vi "Actor Core.vi"(8 "error in":errorcluster, 11 "Image Acquisition in":refnum<class "Image Acquisition.lvclass">) -> (0 "error out":errorcluster, 3 "Actor out":refnum<class "Actor.lvclass">)   [LabVIEW 2016, in "Image Acquisition.lvlib" / "Image Acquisition.lvclass"]
doc: "(<B>Filename</B>: Actor Framework.lvlib:Actor.lvclass:Actor Core.vi)\n\nReceives messages to the actor, reacts to them, and initiates any error handling that may shut the actor down.\n\nDescendant classes may override this VI to append parallel tasks for the actor to complete while it handles messages. Overrides use the Call Parent Method node."
uses:
  Image Acquisition.lvclass
  C:/Program Files (x86)/National Instruments/LabVIEW 2016/vi.lib/ActorFramework/Actor/Actor.lvclass
  <vilib>/ActorFramework/Actor/Actor.lvclass
  Controls/States.ctl
  Controls/Acuisition Actor Data.ctl
  UI/UI/Controls/Start Acquisition.ctl
  <vilib>/userdefined/High Color/IMAQdx.ctl
  <vilib>/ActorFramework/Message Enqueuer/Message Enqueuer.lvclass
  <vilib>/vision/Image Controls.llb/IMAQ Image.ctl
  Image Acquisition.lvclass/Image Acquisition.ctl
  <vilib>/ActorFramework/Actor/Actor.lvclass/Actor.ctl
  <vilib>/ActorFramework/Message Enqueuer/Message Enqueuer.lvclass/Message Enqueuer.ctl
  Image Acquisition Messages/UpdatedMethod Msg/UpdatedImage Msg.lvclass/UpdatedImage Msg.ctl
  <vilib>/ActorFramework/Message Enqueuer/Init from Existing Queue.vi
  <vilib>/ActorFramework/Message Enqueuer/Enqueue.vi
  Image Acquisition Messages/UpdatedMethod Msg/UpdatedImage Msg.lvclass
  C:/Program Files (x86)/National Instruments/LabVIEW 2016/vi.lib/ActorFramework/Message/Message.lvclass
  <vilib>/ActorFramework/Stop Msg/Stop Msg.lvclass
  <vilib>/ActorFramework/Message Priority Queue/Priority Enqueue.vi
  <vilib>/vision/driver/NI_Vision_Acquisition_Software.lvlib
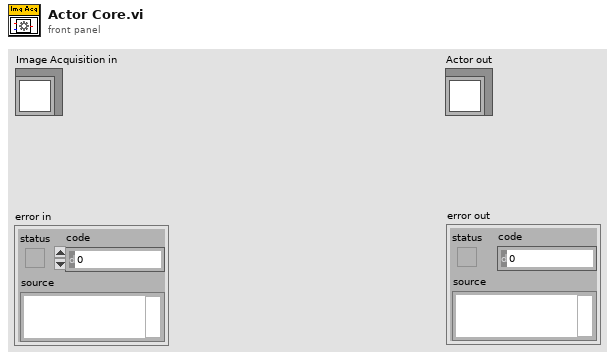
[diagram p1: front panel]
types:
  T1 = typedef "Acuisition Actor Data.ctl" = cluster{"Start Acquisition":T2, "Caller Enqueuer":refnum<class "Message Enqueuer.lvclass">, "Self Enqueuer":refnum<class "Message Enqueuer.lvclass">, "UI Enqueuer":refnum<class "Message Enqueuer.lvclass">, "Image Acquisition in":refnum<class "Image Acquisition.lvclass">, "Target Actor Enqueuer":refnum<class "Message Enqueuer.lvclass">, "Live Session":T3, "Live Image Buffer":T4, "Started?":bool}
  T2 = typedef "Start Acquisition.ctl" = cluster{"Image Indicator Reference":refnum<vi>, "Start":bool, "Camera":T3}
  T3 = typedef "IMAQdx.ctl" = refnum<k21>
  T4 = typedef "IMAQ Image.ctl" = refnum<image>
  T5 = typedef "States.ctl" = enum16{"Poll", "Initialize", "Start Acquisition", "Snap Image", "Stop Acquistion", "Error"}
  T6 = typedef "Image Type" = u32
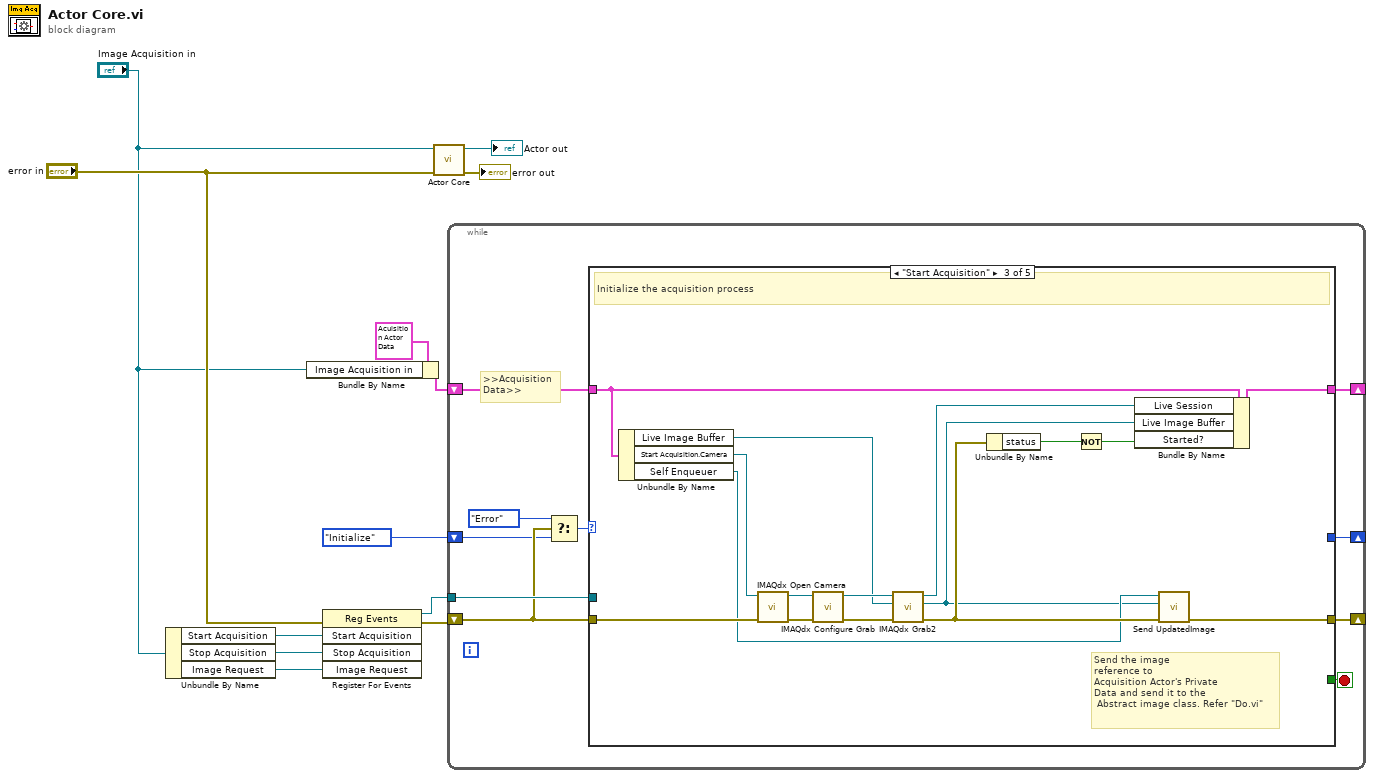
[diagram p0: block diagram]
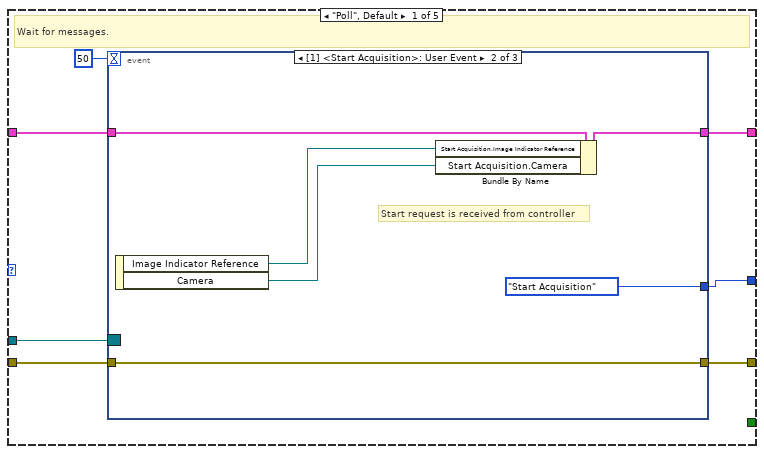
[diagram p2: hidden frame]
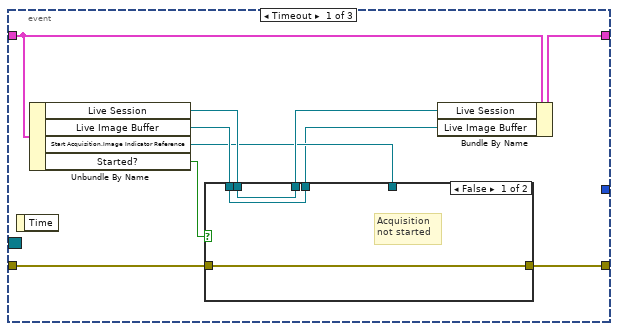
[diagram p3: hidden frame]
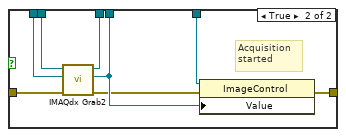
[diagram p4: hidden frame]
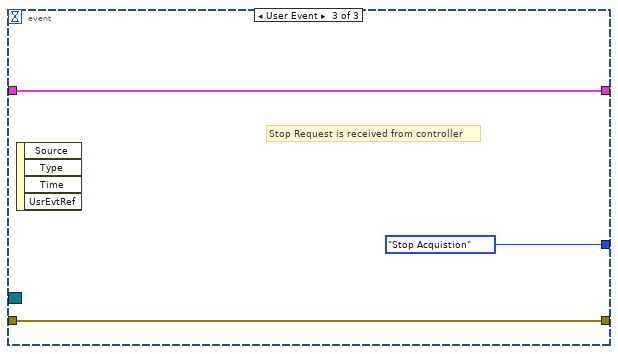
[diagram p5: hidden frame]
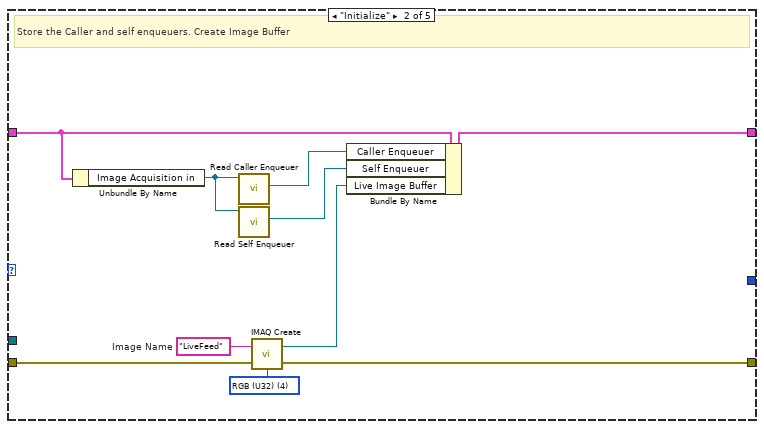
[diagram p6: hidden frame]
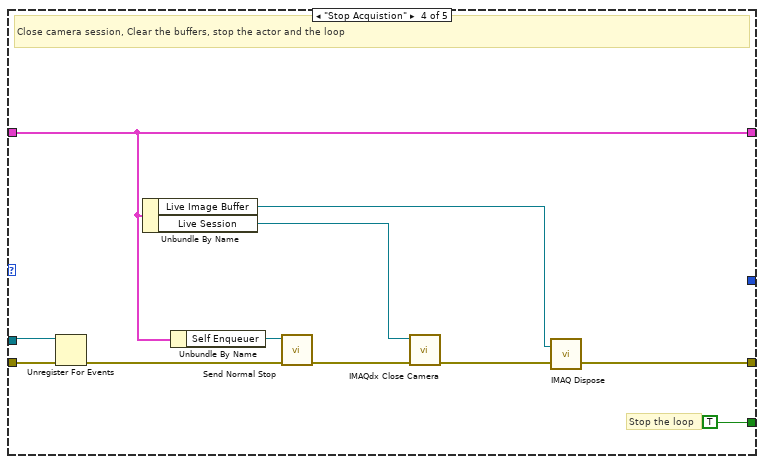
[diagram p7: hidden frame]
diagram:
  n1 = Unbundle By Name("Image Acquisition in") -> ("Start Acquisition"=w3:refnum<user-event>, "Stop Acquisition"=w2:refnum<user-event>, "Image Request"=w1:refnum<user-event>)
  n2 = Bundle By Name(cluster=T1 {"Start Acquisition"={"Image Indicator Reference"=refnum, "Start"=FALSE, "Camera"=""}, "Caller Enqueuer"=refnum, "Self Enqueuer"=refnum, "UI Enqueuer"=refnum, "Image Acquisition in"=refnum, "Target Actor Enqueuer"=refnum, "Live Session"="", "Live Image Buffer"=refnum, "Started?"=FALSE}, "Image Acquisition in"="Image Acquisition in") -> (w8:T1)
  n3 = register-events(error in="error in", w3, w2, w1) -> (reference out=w6:refnum<event-registration>, error out=w7:errorcluster)  [unwired: 1 in]
  n4 = call-parent "Actor Core.vi"("error in"="error in", "Actor in"="Image Acquisition in") -> ("error out"=→"error out":errorcluster, "Actor out"=→"Actor out":refnum<class "Actor.lvclass">)  [unwired: 8 in]
  n5 = while {
    shift-right: [w18] -> _
    shift-left: States."Initialize" -> [w14]
    shift-right: [w21] -> _
    shift-left: w8 -> [w22]
    shift-right: [w20] -> _
    shift-left: w7 -> [w16]
    tunnel: w6 -> [w19]
    stop <- w17 stop-if-true
    # ">>Acquisition\nData>>"
    n6 = Select(t=States."Error", s=w16, f=w14) -> (s? t:f=w13:T5)
    n7 = case shown="\"Start Acquisition\"" w13 {
      tunnel: w22 -> [w28 w69 w85 w93 w98]
      tunnel: [w27 w67 w79 w93 w98] -> w21
      tunnel: [w25 w60 w74 w90 w97] -> w20
      tunnel: w16 -> [w26 w61 w80 w88 w97]
      tunnel: w19 -> [w24 _ _ w86 _]
      tunnel: [w23 _ _ _ _] -> w18
      tunnel: [_ _ _ TRUE _] -> w17
      frame "Poll", Default {
        # "Wait for messages."
        n8 = event shown="[1] <Start Acquisition>: User Event" {
          selector: w24 -> [_ _ _]
          dyn-events: _ -> [_ _ _]
          timeout: 50 -> [_ _ _]
          tunnel: w28 -> [w36 w56 w59]
          tunnel: [w34 w55 w59] -> w27
          tunnel: w26 -> [w39 w51 w57]
          tunnel: [w32 w51 w57] -> w25
          tunnel: [_ States."Start Acquisition" States."Stop Acquistion"] -> w23
          event Timeout {
            n9 = event-data() -> ()  [unwired: 1 in, 1 out]
            n10 = Unbundle By Name(w36) -> ("Live Session"=w38:T3, "Live Image Buffer"=w37:T4, "Start Acquisition.Image Indicator Reference"=w33:refnum<vi>, "Started?"=w31:bool)
            n11 = case shown="False" w31 {
              tunnel: w39 -> [w40 w50]
              tunnel: w38 -> [w42 w49]
              tunnel: w37 -> [w41 w48]
              tunnel: [w42 w47] -> w35
              tunnel: w33 -> [_ w46]
              tunnel: [w41 w45] -> w30
              tunnel: [w40 w43] -> w32
              frame False {
                # "Acquisition \nnot started"
              }
              frame True {
                # "Acquisition \nstarted"
                n12 = call <vilib>:"IMAQdx Grab2.vi"("error in"=w50, "Image In"=w48, "Session In"=w49) -> ("error out"=w44:errorcluster, "Image Out"=w45:T4, "Session Out"=w47:T3)  [unwired: 5 in, 1 out]
                n13 = property class="ImageControl"(reference=w46, error in=w44, "Value"=w45) -> (error out=w43:errorcluster)  [unwired: 1 out]
              }
            }
            n14 = Bundle By Name(cluster=w36, "Live Session"=w35, "Live Image Buffer"=w30) -> (w34:T1)
          }
          event User Event {
            # "Start request is received from controller"
            n15 = event-data() -> ("Image Indicator Reference"=w54:refnum<vi>, "Camera"=w53:T3)  [unwired: 1 in]
            n16 = Bundle By Name(cluster=w56, "Start Acquisition.Image Indicator Reference"=w54, "Start Acquisition.Camera"=w53) -> (w55:T1)
          }
          event User Event {
            # "Stop Request is received from controller"
            n17 = event-data() -> ()  [unwired: 1 in, 4 out]
          }
        }
      }
      frame "Initialize" {
        w64 = T6 4 items=["Grayscale (U8)", "Grayscale (I16)", "Grayscale (SGL)", "Complex (CSG)", "RGB (U32)", "HSL (U32)", "RGB (U64)", "Grayscale (U16)"] ("Image Type")
        w63 = "LiveFeed"  # Image Name
        # "Store the Caller and self enqueuers. Create Image Buffer"
        n18 = Unbundle By Name(w69) -> ("Image Acquisition in"=w68:refnum<class "Image Acquisition.lvclass">)
        n19 = call <vilib>:"Read Caller Enqueuer.vi"("Actor"=w68) -> ("Caller Enqueuer"=w66:refnum<class "Message Enqueuer.lvclass">)  [unwired: 10 in]
        n20 = call <vilib>:"Read Self Enqueuer.vi"("Actor"=w68) -> ("Self Enqueuer"=w65:refnum<class "Message Enqueuer.lvclass">)  [unwired: 10 in]
        n21 = call "IMAQ Create"("Image Name"=w63, "Image Type"=w64, "error in (no error)"=w61) -> ("New Image"=w62:T4, "error out"=w60:errorcluster)  [unwired: 2 in]
        n22 = Bundle By Name(cluster=w69, "Caller Enqueuer"=w66, "Self Enqueuer"=w65, "Live Image Buffer"=w62) -> (w67:T1)
      }
      frame "Start Acquisition" {
        # "Send the image \nreference to \nAcquisition Actor's Private\nData and send it to the\n Abstract image class. Refer \"Do.vi\""
        # "Initialize the acquisition process"
        n23 = Unbundle By Name(w85) -> ("Live Image Buffer"=w70:T4, "Start Acquisition.Camera"=w84:T3, "Self Enqueuer"=w73:refnum<class "Message Enqueuer.lvclass">)
        n24 = call <vilib>:"IMAQdx Open Camera.vi"("error in"=w80, "Session In"=w84) -> ("error out"=w83:errorcluster, "Session Out"=w82:T3)  [unwired: 8 in]
        n25 = call <vilib>:"IMAQdx Configure Grab.vi"("error in"=w83, "Session In"=w82) -> ("error out"=w71:errorcluster, "Session Out"=w81:T3)  [unwired: 8 in]
        n26 = call <vilib>:"IMAQdx Grab2.vi"("error in"=w71, "Image In"=w70, "Session In"=w81) -> ("error out"=w75:errorcluster, "Image Out"=w72:T4, "Session Out"=w78:T3)  [unwired: 5 in, 1 out]
        n27 = Unbundle By Name(w75) -> ("status"=w77:bool)
        n28 = Not(x=w77) -> (.not. x?=w76:bool)
        n29 = Bundle By Name(cluster=w85, "Live Session"=w78, "Live Image Buffer"=w72, "Started?"=w76) -> (w79:T1)
        n30 = call "Send UpdatedImage.vi"("error in (no error)"=w75, "Image"=w72, "Message Enqueuer"=w73) -> ("error out"=w74:errorcluster)  [unwired: 7 in, 1 out]
      }
      frame "Stop Acquistion" {
        # "Stop the loop"
        # "Close camera session, Clear the buffers, stop the actor and the loop"
        n31 = Unregister For Events(event registration refnum=w86, error in=w88) -> (error out=w87:errorcluster)
        n32 = Unbundle By Name(w93) -> ("Live Image Buffer"=w89:T4, "Live Session"=w92:T3)
        n33 = Unbundle By Name(w93) -> ("Self Enqueuer"=w95:refnum<class "Message Enqueuer.lvclass">)
        n34 = call <vilib>:"Send Normal Stop.vi"("error in (no error)"=w87, "Message Enqueuer"=w95) -> ("error out"=w94:errorcluster)  [unwired: 9 in]
        n35 = call <vilib>:"IMAQdx Close Camera.vi"("error in"=w94, "Session In"=w92) -> ("error out"=w91:errorcluster)  [unwired: 9 in]
        n36 = call "IMAQ Dispose"("Image"=w89, "error in (no error)"=w91) -> ("error out"=w90:errorcluster)  [unwired: 4 in]
      }
      frame "Error" {
      }
    }
  }
